vi "Configure Output.vi"(7 "Enable Output (T: Enable)":bool=TRUE, 8 "error in (no error)":errorcluster, 9 "Voltage Level (0.0 V)":dbl caption="Voltage Level (0 V)" format="%.2f", 10 "Channel (0: +6V Channel)":i32(ring) caption="Channel (0: +6V)" items=["+6V Channel", "+25V Channel", "-25V Channel"], 11 "VISA resource name":refnum<visa-resource-name>) -> (0 "error out":errorcluster, 3 "VISA resource name out":refnum<visa-resource-name>)   [LabVIEW 2020, in "RIGOL DP1000 Series.lvlib"]
doc: "Configures output voltage level, channel, and enables or disables the output of the power supply."
uses:
  <instrlib>/RIGOL DP1000 Series/RIGOL DP1000 Series.lvlib
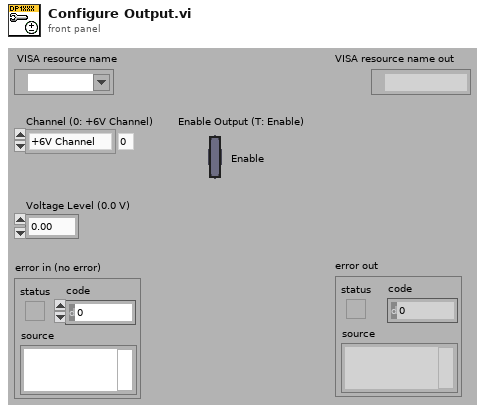
[diagram p1: front panel]
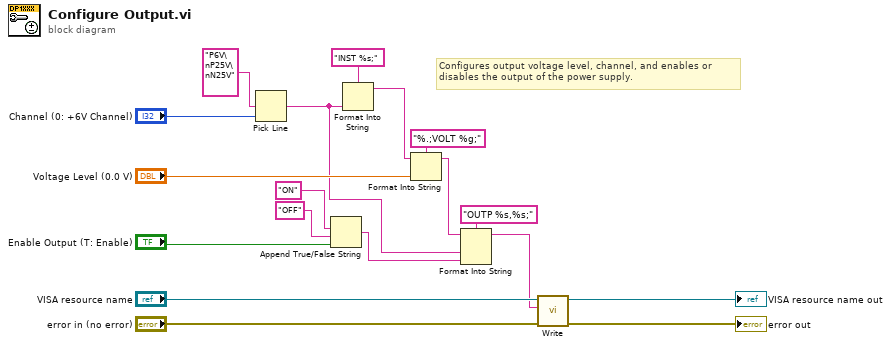
[diagram p0: block diagram]
diagram:
  # "Configures output voltage level, channel, and enables or \ndisables the output of the power supply."
  n1 = Pick Line(multi-line string="P6V\nP25V\nN25V", line index="Channel (0: +6V Channel)") -> (output string=w7:string)  [unwired: 1 out]
  n2 = Append True/False String(1:"Enable Output (T: Enable)", 2:"OFF", 3:"ON") -> (0:w10:string)  [unwired: 1 out]
  n3 = Format Into String(format string="INST %s;", w7) -> (resulting string=w6:string)  [unwired: 2 in, 1 out]
  n4 = Format Into String(format string="%.;VOLT %g;", initial string=w6, "Voltage Level (0.0 V)") -> (resulting string=w12:string)  [unwired: 1 in, 1 out]
  n5 = Format Into String(format string="OUTP %s,%s;", initial string=w12, w7, w10) -> (resulting string=w1:string)  [unwired: 1 in, 1 out]
  n6 = call <instrlib>:"Write.vi"("error in (no error)"="error in (no error)", "Write Buffer (\"\")"=w1, "VISA resource name"="VISA resource name") -> ("error out"=→"error out":errorcluster, "VISA resource name out"=→"VISA resource name out":refnum<visa-resource-name>)  [unwired: 7 in]
